vi "C37 Read Next Frame.vi"(8 "error in (no error)":errorcluster, 10 "Timeout [ms]":i32, 11 "Pseudo PDC ID":i32) -> (0 "error out":errorcluster)   [LabVIEW 2013, in "C37118-DLL.lvlib"]
uses:
  C37118-DLL.lvlib
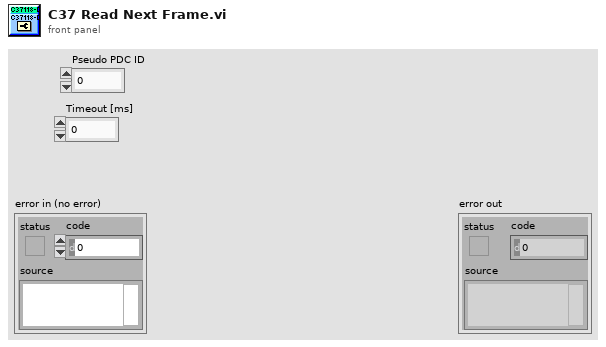
[diagram p1: front panel]
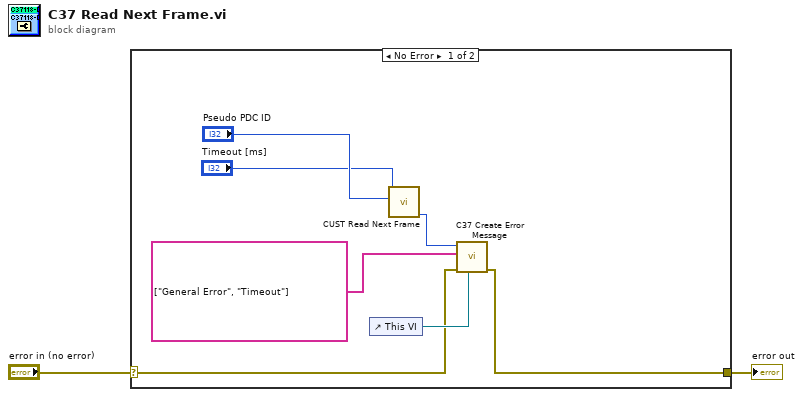
[diagram p0: block diagram]
diagram:
  n1 = case shown="No Error" "error in (no error)" {
    selector: "error in (no error)" -> [w8 w10]
    tunnel: [w7 w10] -> w2
    frame No Error {
      n2 = control-ref of="This VI"() -> (w9:refnum<vi>)
      n3 = call "CUST Read Next Frame.vi"("pseudoPdcId"="Pseudo PDC ID", "timeoutMs"="Timeout [ms]") -> ("function return"=w3:i32)  [unwired: 9 in]
      n4 = call "C37 Create Error Message.vi"("VI Reference"=w9, "error in (no error)"=w8, "Error Messages"=string[] ["General Error", "Timeout"], "function return"=w3) -> ("error out"=w7:errorcluster)  [unwired: 7 in]
    }
    frame Error {
    }
  }
  "error out" <- w2
